vi "get_left_right_distance.vi"(11 "NXT":T1={"Hardware"="NXT", "Flattened String"=""}) -> (0 "right distance":dbl, 1 "left distance":dbl, 3 "NXT 2":T1={"Hardware"="NXT", "Flattened String"=""})   [LabVIEW 2012]
uses:
  <vilib>/NXT/Subs/LVHSConnector.ctl
  <vilib>/NXT/Subs/MotorOutput.ctl
  <vilib>/NXT/Dual Mode Library/Motors/MotorReverse.vi
  <vilib>/NXT/Dual Mode Library/Motors/MotorBrake.vi
  <vilib>/NXT/Dual Mode Library/Motors/MotorOn.vi
  <vilib>/NXT/Dual Mode Library/prims/addArrayElements_int.vi
  <vilib>/NXT/Dual Mode Library/Waits/Wait_Num(msec).vi
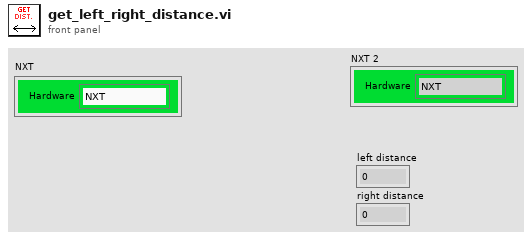
[diagram p1: front panel]
types:
  T1 = typedef "LVHSConnector.ctl" = cluster{"Hardware":string, "Flattened String":string}
  T2 = typedef "MotorOutput.ctl" = u8
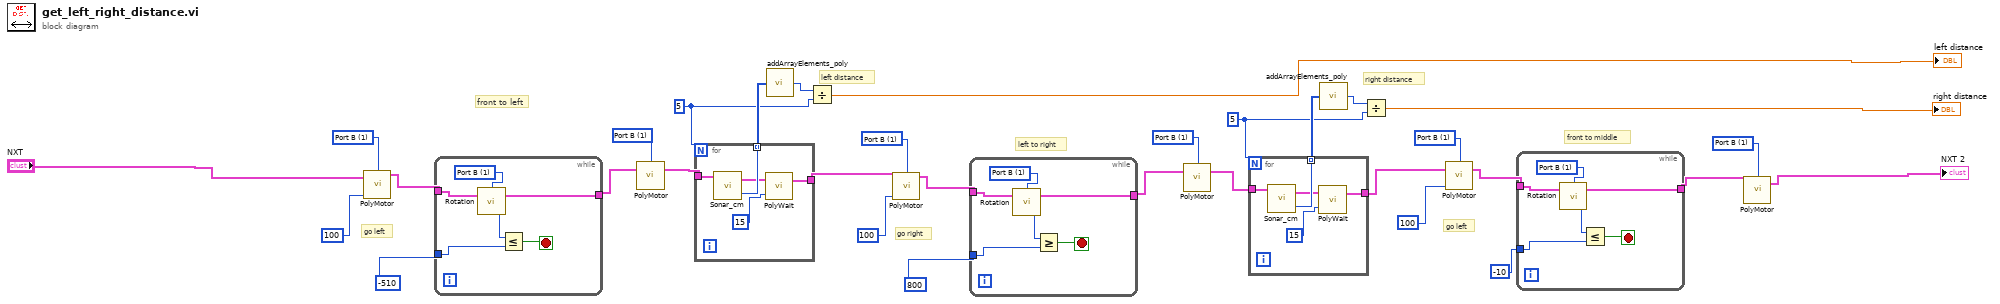
[diagram p0: block diagram]
diagram:
  w3 = 5
  w6 = 5
  w15 = T2 1 items=["Port A"=0, "Port B"=1, "Port C"=2, "Ports A & B"=4, "Ports A & C"=5, "Ports B & C"=6, "All Ports"=3] ("Output Port (All Ports)")
  w16 = T2 1 items=["Port A"=0, "Port B"=1, "Port C"=2, "Ports A & B"=4, "Ports A & C"=5, "Ports B & C"=6, "All Ports"=3] ("Output Port (All Ports)")
  w20 = T2 1 items=["Port A"=0, "Port B"=1, "Port C"=2, "Ports A & B"=4, "Ports A & C"=5, "Ports B & C"=6, "All Ports"=3] ("Output Port (All Ports)")
  w21 = T2 1 items=["Port A"=0, "Port B"=1, "Port C"=2, "Ports A & B"=4, "Ports A & C"=5, "Ports B & C"=6, "All Ports"=3] ("Output Port (All Ports)")
  w25 = T2 1 items=["Port A"=0, "Port B"=1, "Port C"=2, "Ports A & B"=4, "Ports A & C"=5, "Ports B & C"=6, "All Ports"=3] ("Output Port (All Ports)")
  w26 = T2 1 items=["Port A"=0, "Port B"=1, "Port C"=2, "Ports A & B"=4, "Ports A & C"=5, "Ports B & C"=6, "All Ports"=3] ("Output Port (All Ports)")
  # "right distance"
  # "left distance"
  # "go right"
  # "go left"
  # "front to middle"
  # "left to right"
  # "go left"
  # "front to left"
  n1 = call-poly <vilib>:"PolyMotor.vi"("Power (75)"=100, "NXT"="NXT", "Output Port (All Ports)"=w26) -> ("NXT"=w27:T1)  [unwired: 1 in]
  n2 = while {
    tunnel: -510 -> [w37]
    tunnel: w27 -> [w35]
    tunnel: [w34] -> w24
    stop <- w33 stop-if-true
    w36 = T2 1 items=["Port A"=0, "Port B"=1, "Port C"=2, "Ports A & B"=4, "Ports A & C"=5, "Ports B & C"=6, "All Ports"=3] ("Output Port (All Ports)")
    n3 = call <vilib>:"Rotation.vi"("NXT"=w35, "Port (Port A)"=w36) -> ("Angle of Rotation"=w38:i32, "NXT"=w34:T1)  [unwired: 1 in]
    n4 = Less Or Equal?(x=w38, y=w37) -> (x <= y?=w33:bool)
  }
  n5 = call-poly <vilib>:"PolyMotor.vi"("NXT"=w24, "Port (All Ports)"=w25) -> ("NXT"=w10:T1)  [unwired: 2 in]
  n6 = for {
    N: w6 -> [_]
    tunnel: w10 -> [w42]
    tunnel: [w43] -> w8 mode=indexing
    tunnel: [w40] -> w9
    n7 = call <vilib>:"Sonar_cm.vi"("NXT"=w42) -> ("Distance (cm)"=w43:i16, "NXT"=w41:T1)  [unwired: 2 in]
    n8 = call-poly <vilib>:"PolyWait.vi"("Time (100 msec)"=15, "NXT"=w41) -> ("NXT"=w40:T1)  [unwired: 2 in]
  }
  n9 = call-poly <vilib>:"addArrayElements_poly.vi"("Numeric Array"=w8) -> ("Sum"=w7:i32)
  n10 = Divide(x=w7, y=w6) -> (x/y=→"left distance":dbl)
  n11 = call-poly <vilib>:"PolyMotor.vi"("Power (75)"=100, "NXT"=w9, "Output Port (All Ports)"=w21) -> ("NXT"=w22:T1)  [unwired: 1 in]
  n12 = while {
    tunnel: 800 -> [w48]
    tunnel: w22 -> [w46]
    tunnel: [w45] -> w19
    stop <- w44 stop-if-true
    w47 = T2 1 items=["Port A"=0, "Port B"=1, "Port C"=2, "Ports A & B"=4, "Ports A & C"=5, "Ports B & C"=6, "All Ports"=3] ("Output Port (All Ports)")
    n13 = call <vilib>:"Rotation.vi"("NXT"=w46, "Port (Port A)"=w47) -> ("Angle of Rotation"=w49:i32, "NXT"=w45:T1)  [unwired: 1 in]
    n14 = Greater Or Equal?(x=w49, y=w48) -> (x >= y?=w44:bool)
  }
  n15 = call-poly <vilib>:"PolyMotor.vi"("NXT"=w19, "Port (All Ports)"=w20) -> ("NXT"=w2:T1)  [unwired: 2 in]
  n16 = for {
    N: w3 -> [_]
    tunnel: w2 -> [w53]
    tunnel: [w54] -> w5 mode=indexing
    tunnel: [w51] -> w1
    n17 = call <vilib>:"Sonar_cm.vi"("NXT"=w53) -> ("Distance (cm)"=w54:i16, "NXT"=w52:T1)  [unwired: 2 in]
    n18 = call-poly <vilib>:"PolyWait.vi"("Time (100 msec)"=15, "NXT"=w52) -> ("NXT"=w51:T1)  [unwired: 2 in]
  }
  n19 = call-poly <vilib>:"addArrayElements_poly.vi"("Numeric Array"=w5) -> ("Sum"=w4:i32)
  n20 = Divide(x=w4, y=w3) -> (x/y=→"right distance":dbl)
  n21 = call-poly <vilib>:"PolyMotor.vi"("Power (75)"=100, "NXT"=w1, "Output Port (All Ports)"=w16) -> ("NXT"=w17:T1)  [unwired: 1 in]
  n22 = while {
    tunnel: -10 -> [w59]
    tunnel: w17 -> [w57]
    tunnel: [w56] -> w14
    stop <- w55 stop-if-true
    w58 = T2 1 items=["Port A"=0, "Port B"=1, "Port C"=2, "Ports A & B"=4, "Ports A & C"=5, "Ports B & C"=6, "All Ports"=3] ("Output Port (All Ports)")
    n23 = call <vilib>:"Rotation.vi"("NXT"=w57, "Port (Port A)"=w58) -> ("Angle of Rotation"=w60:i32, "NXT"=w56:T1)  [unwired: 1 in]
    n24 = Less Or Equal?(x=w60, y=w59) -> (x <= y?=w55:bool)
  }
  n25 = call-poly <vilib>:"PolyMotor.vi"("NXT"=w14, "Port (All Ports)"=w15) -> ("NXT"=→"NXT 2":T1)  [unwired: 2 in]
